vi "Handle Error.vi"(8 "error in (no error)":errorcluster, 11 "State Machine in":refnum<class "State Machine.lvclass">) -> (0 "error out":errorcluster, 2 "stop actor?":bool=TRUE, 3 "State Machine out":refnum<class "State Machine.lvclass">)   [LabVIEW 2024, in "State Machine.lvlib" / "State Machine.lvclass"]
doc: "<p>(<strong>Filename</strong>: <span class=\"dnl\">Actor Framework.lvlib:Actor.lvclass:Handle Error.vi</span>)</p>\n<p>Defines how the actor handles an error that occurred while processing a message. By default, this method does nothing except stop the actor.</p>"
uses:
  State Machine.lvclass
  State Machine.lvclass/State Machine.ctl
  <vilib>/ActorFramework/Actor/Actor.lvclass
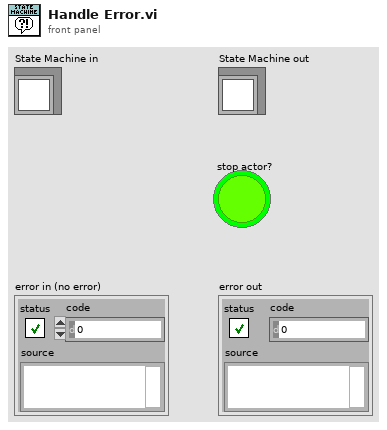
[diagram p1: front panel]
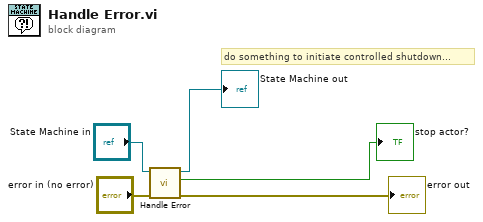
[diagram p0: block diagram]
diagram:
  # "do something to initiate controlled shutdown..."
  n1 = call-parent "Handle Error.vi"("error in (no error)"="error in (no error)", "Actor in"="State Machine in") -> ("error out"=→"error out":errorcluster, "stop actor?"=→"stop actor?":bool, "Actor out"=→"State Machine out":refnum<class "State Machine.lvclass">)  [unwired: 7 in]
